vi "2_project_main.vi"() -> ()   [LabVIEW 2014]
uses:
  <vilib>/Math Plots/3D Math Plots/3D Surface/3D Surface XCtrl/3D Surface.xctl
  <vilib>/Math Plots/3D Math Plots/3D Surface/3D Surface Datatype/Public/Plot Helper (Vector).vi
  <vilib>/Utility/file.llb/Write To Spreadsheet File (DBL).vi
  <vilib>/Analysis/Matrix/Numeric/Conversions/Matrix To Array - RM.vi
  array_Global 2.vi
  <vilib>/Math Plots/3D Math Plots/3D Surface/3D Surface Datatype/3D Surface Datatype.lvclass
  <vilib>/Analysis/Matrix/NI_Matrix.lvlib
  <vilib>/ptbypt/NI_PtbyPt.lvlib
panel:
  in  "Tab Control":enum32{"Signal plot", "Matrix function"}(tab)
  in  "Path":path
  out "Intensity Graph":dbl[][](graph)
  out "3D Surface":refnum<class "3D Plot Datatype.lvclass">[](xcontrol)
  out "output file refnum":refnum<file>
  out "appended array":dbl[][][](array[numeric])
  in  "element":dbl[](array[knob]) scale=0.0..300.0
  in  "element 2":dbl[](array[knob]) scale=0.0..300.0
  in  "stop":bool
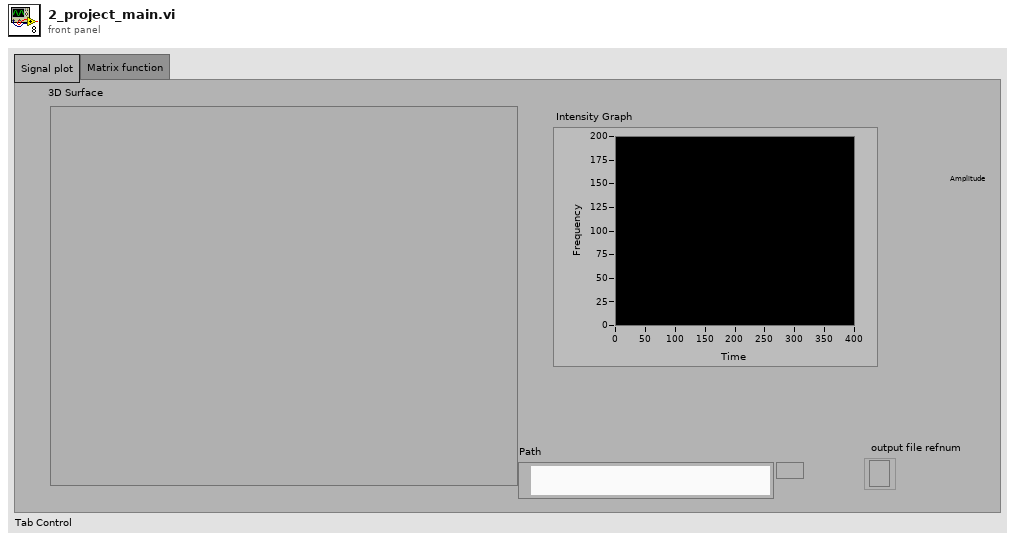
[diagram p1: front panel]
types:
  T1 = typedef "NI_Matrix.lvlib/RealMatrix.ctl" = dbl[][]
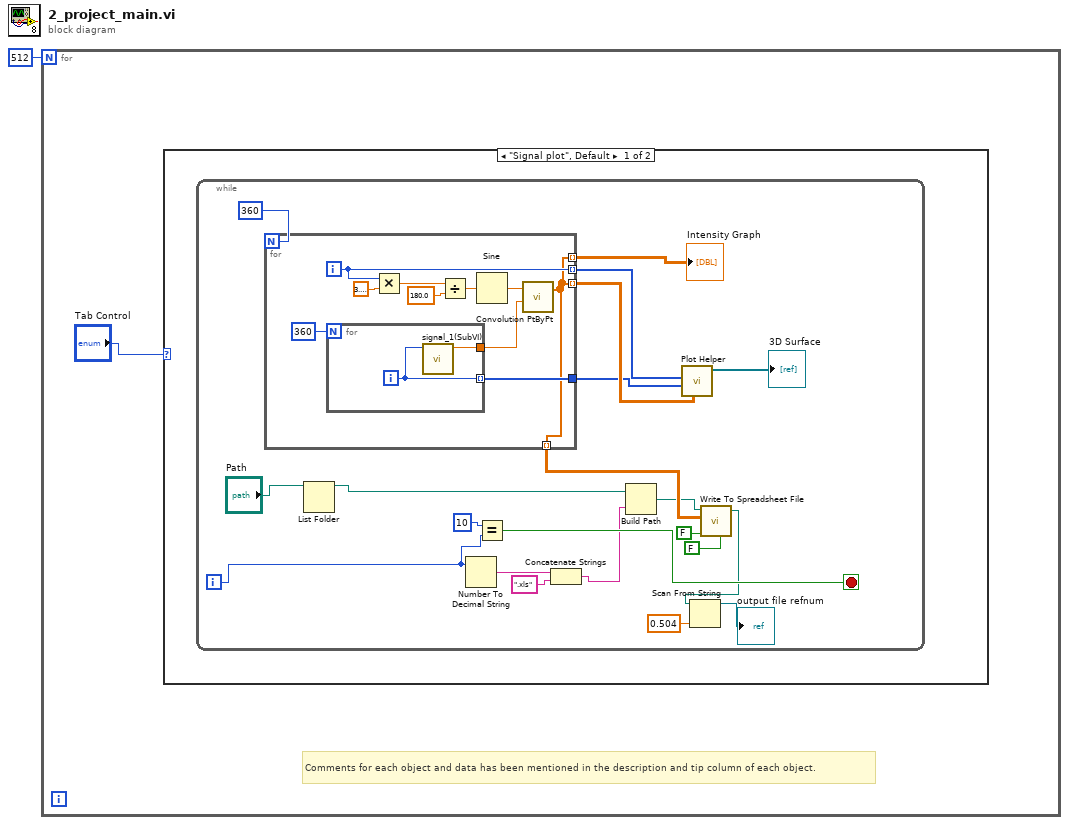
[diagram p0: block diagram]
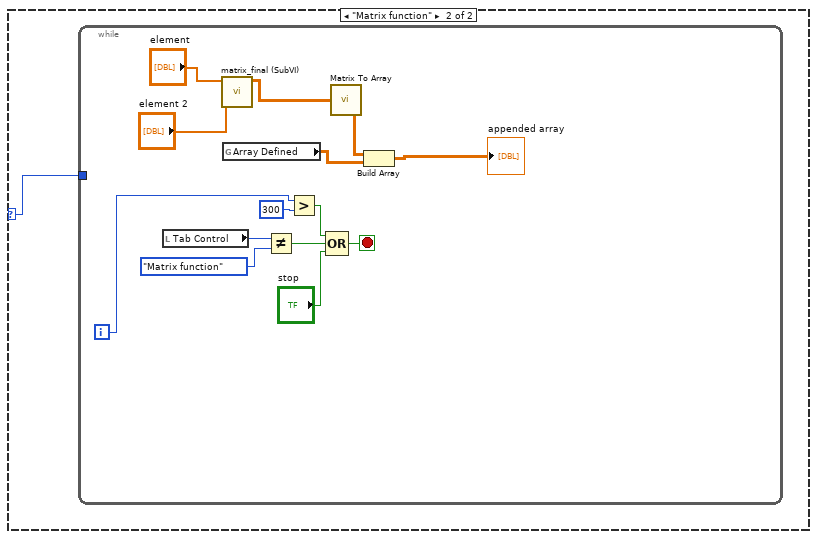
[diagram p2: hidden frame]
diagram:
  n1 = for {
    N: 512 -> [_]
    # "Comments for each object and data has been mentioned in the description and tip column of each object."
    n2 = case shown="\"Signal plot\", Default" "Tab Control" {
      selector: "Tab Control" -> [_ w36]
      frame "Signal plot", Default {
        n3 = while {
          i -> [w8]
          stop <- w10 stop-if-true
          n4 = for {
            N: 360 -> [_]
            tunnel: [w29] -> w19 mode=indexing
            tunnel: [w24] -> w21 mode=indexing
            tunnel: [w32] -> w20
            tunnel: [w24] -> w18 mode=indexing
            tunnel: [w24] -> w14 mode=indexing
            i -> [w29]
            n5 = for {
              N: 360 -> [_]
              tunnel: [w35] -> w25
              tunnel: [w34] -> w32 mode=indexing
              i -> [w34]
              n6 = call "signal_1(SubVI).vi"("x"=w34) -> ("Numeric"=w35:dbl)  [unwired: 10 in]
            }
            n7 = Multiply(x=w29, y=3.141592653589793) -> (x*y=w27:dbl)
            n8 = Divide(x=w27, y=180.0) -> (x/y=w31:dbl)
            n9 = Sine(x=w31) -> (sin(x)=w26:dbl)
            n10 = call <vilib>:"Convolution PtByPt.vi"("x"=w26, "y"=w25) -> ("X*Y"=w24:dbl[])  [unwired: 3 in, 1 out]
          }
          "Intensity Graph" <- w18
          n11 = List Folder(path="Path") -> (path out=w15:path)  [unwired: 3 in, 3 out]
          n12 = Number To Decimal String(number=w8) -> (decimal integer string=w12:string)  [unwired: 1 in]
          n13 = Equal?(x=10, y=w8) -> (x = y?=w10:bool)
          n14 = Concatenate Strings(w12, ".xls" ("string")) -> (w9:string)
          n15 = Build Path(base path=w15, name or relative path=w9) -> (appended path=w7:path)
          n16 = call-poly <vilib>:"Plot Helper.vi"("z matrix"=w21, "y vector"=w20, "x vector"=w19) -> ("3D Plot lvclass Array out"=→"3D Surface":refnum<class "3D Plot Datatype.lvclass">[])  [unwired: 3 in, 5 out]
          n17 = call-poly <vilib>:"Write To Spreadsheet File.vi"("transpose? (no:F)"=FALSE, "append to file? (new file:F)"=FALSE, "2D data"=w14, "file path (dialog if empty)"=w7) -> ("new file path (Not A Path if cancelled)"=w4:path)  [unwired: 4 in]
          n18 = Scan From String(w4, default 1=0.504 ("default value 1")) -> (→"output file refnum":refnum<file>)  [unwired: 3 in, 1 out]
        }
      }
      frame "Matrix function" {
        n19 = while {
          tunnel: w36 -> [_]
          i -> [w44]
          stop <- w45 stop-if-true
          n20 = local read "Tab Control"() -> (w41:enum32{"Signal plot", "Matrix function"})
          n21 = call "matrix_final (SubVI).vi"("element 2"="element 2", "element"="element") -> ("Real Matrix"=w39:T1)  [unwired: 9 in]
          n22 = global read "array_Global 2.vi" "Array Defined"() -> (w49:dbl[][])
          n23 = Not Equal?(x=w41, y=enum32{"Signal plot", "Matrix function"}."Matrix function" ("Tab Control")) -> (x != y?=w47:bool)
          n24 = Greater?(x=w44, y=300) -> (0:w42:bool)
          n25 = Compound Arithmetic op=OR(w42, w47, "stop") -> (w45:bool)
          n26 = call-poly <vilib>:"Matrix To Array.vi"("Real Matrix"=w39) -> ("Real 2D Array"=w50:dbl[][])
          n27 = Build Array(w50, w49) -> (→"appended array":dbl[][][])
        }
      }
    }
  }
